vi "禹山浊度_获取温度和测量值.vi"(8 "error in (no error)":errorcluster caption="错误输入（无错误）", 11 "MB session in":refnum<class "MB_Master.lvclass">) -> (0 "error out":errorcluster caption="错误输出", 2 "输出值":cluster{"温度测量值":sgl, "浊度":sgl}, 3 "MB session out":refnum<class "MB_Master.lvclass">)   [LabVIEW 2016, in "斯坦道多参数.lvlib"]
uses:
  <vilib>/Plasmionique/MB Master/MB_Master/MB_Master.lvclass
  <vilib>/Plasmionique/MB Master/MB Master.lvlib
  <vilib>/ptbypt/NI_PtbyPt.lvlib
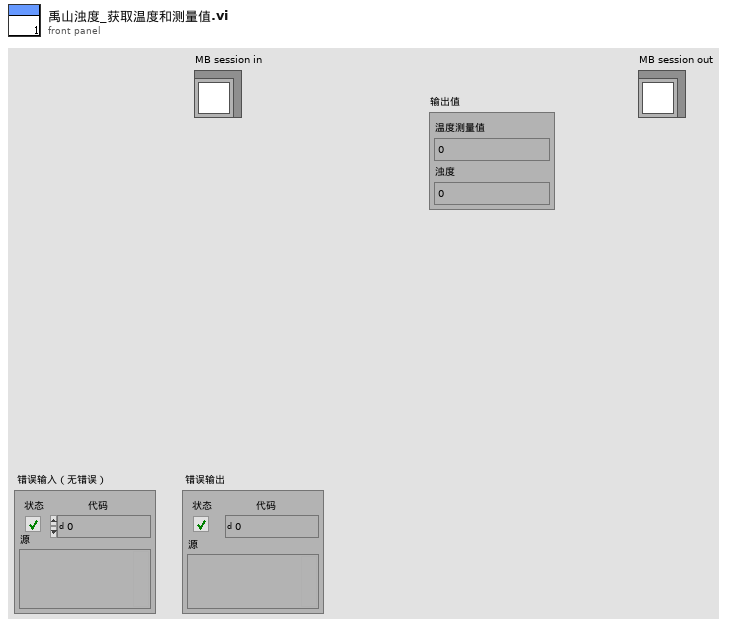
[diagram p1: front panel]
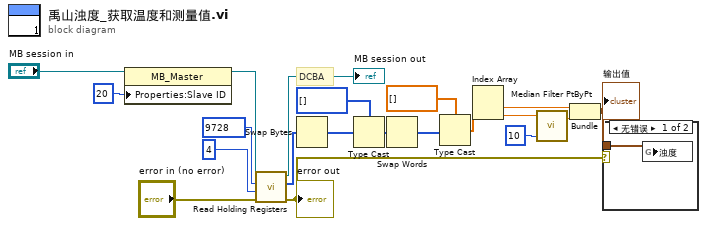
[diagram p0: block diagram]
diagram:
  # "DCBA"
  n1 = property class="MB_Master"(reference="MB session in", "Properties:Slave ID"=u16 20 ("y")) -> (reference out=w12:refnum<class "MB_Master.lvclass">)  [unwired: 1 in, 1 out]
  n2 = call <vilib>:"Read Holding Registers.vi"("error in (no error)"="error in (no error)", "quantity"=u16 4, "starting address"=u16 9728, "MB session in"=w12) -> ("error out"=w7:errorcluster, "Registers"=w10:u16[], "MB session out"=→"MB session out":refnum<class "MB_Master.lvclass">)  [unwired: 5 in]
  "error out" <- w7
  n3 = Swap Bytes(anything=w10) -> (byte swapped=w9:u16[])
  n4 = Type Cast(type=u32[] [] ("数组 2"), x=w9) -> (*(type *) &x=w16:u32[])
  n5 = Swap Words(1:w16) -> (0:w18:u32[])
  n6 = Type Cast(type=sgl[] [] ("数组 2"), x=w18) -> (*(type *) &x=w14:sgl[])
  n7 = Index Array(array=w14) -> (element #1=w8:sgl, element #2=w2:sgl)  [unwired: 2 in]
  n8 = call <vilib>:"Median Filter PtByPt.vi"("rank"=10, "x"=w2) -> ("Filtered x"=w1:dbl)  [unwired: 2 in, 1 out]
  n9 = Bundle("数值"=w8, "Filtered x"=w1) -> (w6:cluster{"数值":sgl, "Filtered x":dbl})  [unwired: 1 in]
  "输出值" <- w6
  n10 = case shown="无错误" w7 {
    tunnel: w6 -> [w21 _]
    frame No Error {
      n11 = global write "禹山过程全局变量.vi" "浊度"(w21) -> ()
    }
    frame Error {
    }
  }
